vi "if_v1_v0.vi"() -> ()   [LabVIEW 2010]
panel:
  in  "Selectie":bool=TRUE
  in  "Numeric 2":u8=170
  in  "Numeric":u8=85
  out "Array":bool[](array[boolean])=[TRUE, FALSE, TRUE, FALSE, TRUE, FALSE, TRUE, FALSE]
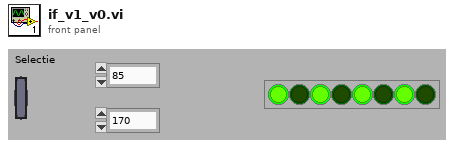
[diagram p1: front panel]
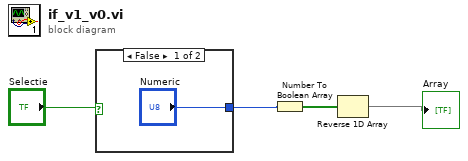
[diagram p0: block diagram]
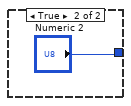
[diagram p2: hidden frame]
diagram:
  n1 = case shown="False" "Selectie" {
    tunnel: ["Numeric" "Numeric 2"] -> w1
    frame False {
    }
    frame True {
    }
  }
  n2 = Number To Boolean Array(number=w1) -> (Boolean array=w4:bool[])
  n3 = Reverse 1D Array(array=w4) -> (reversed array=→"Array":bool[])
